vi "C-Scan - Reverse B-Scan.vi"(7 "Micropulse # In":i32, 8 "Define C-Scan Index":T1={"Index Start"=0.0, "Index Length"=260.0, "Indexing\nResolution"=5.0, "Ch1 Start"=0.0, "Ch1 Finish"=0.0, "Ch2 Start"=0.0, "Ch2 Finish"=0.0} {"Ch2 Finish" format="%#_6f"; "Ch2 Start" format="%#_6f"; "Ch1 Finish" format="%#_6f"; "Ch1 Start" format="%#_6f"; "Index Start" format="%#_6f"; "Index Length" format="%#_6f"; "Indexing\nResolution" format="%#_6f"}, 9 "FLZ Scan definition":T2={"Scan Start"=0.0, "Scan Length"=280.0, "Inspection Resolution"=0.5, "Direction"=enum."Forwards"} {"Inspection Resolution" format="%#_6f"; "Scan Start" format="%#_6f"; "Scan Length" format="%#_6f"}, 10 "C-Scan In Progress?":bool, 11 "B-Scan In Progress?":bool) -> (3 "B-Scan Just Finished?":bool)   [LabVIEW 2026, in "MicroPulse_Driver.lvlib"]
uses:
  MicroPulse_Driver.lvlib
  Data/Datatypes/MP - fly scan range.ctl
  Data/Datatypes/MP - inspection direction.ctl
  Data/Datatypes/MP - C-Scan Definition.ctl
  Low Level/FGV - B-Scan Active - Action [Enum].ctl
  <instrlib>/Micropulse/Micropulse.lvlib
panel:
  # "C-Scan Index"
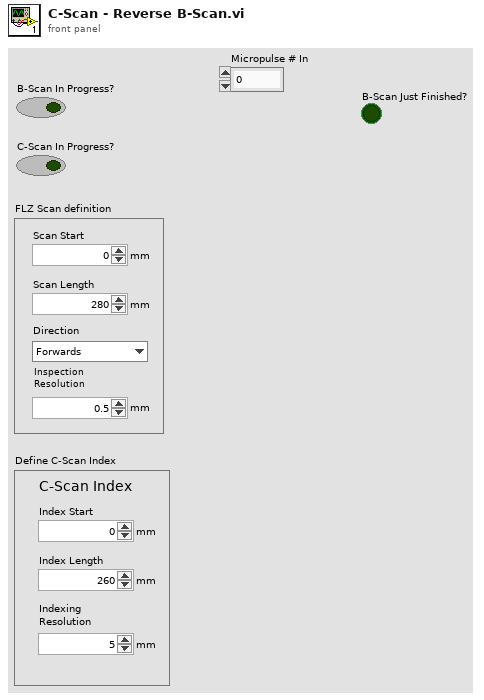
[diagram p1: front panel]
types:
  T1 = typedef "Micropulse.lvlib/MP - C-Scan Definition.ctl" = cluster{"Index Start":dbl, "Index Length":dbl, "Indexing\nResolution":dbl, "Ch1 Start":dbl, "Ch1 Finish":dbl, "Ch2 Start":dbl, "Ch2 Finish":dbl}
  T2 = typedef "Micropulse.lvlib/MP - fly scan range.ctl" = cluster{"Scan Start":dbl, "Scan Length":dbl, "Inspection Resolution":dbl, "Direction":T3}
  T3 = typedef "Micropulse.lvlib/MP - inspection direction.ctl" = enum16{"Forwards", "Backwards"}
  T4 = typedef "MicroPulse_Driver.lvlib/FGV - B-Scan Active - Action [Enum].ctl" = enum16{"Read", "Read & Reset Start Flag", "Start B-Scan", "B-Scan Finished"}
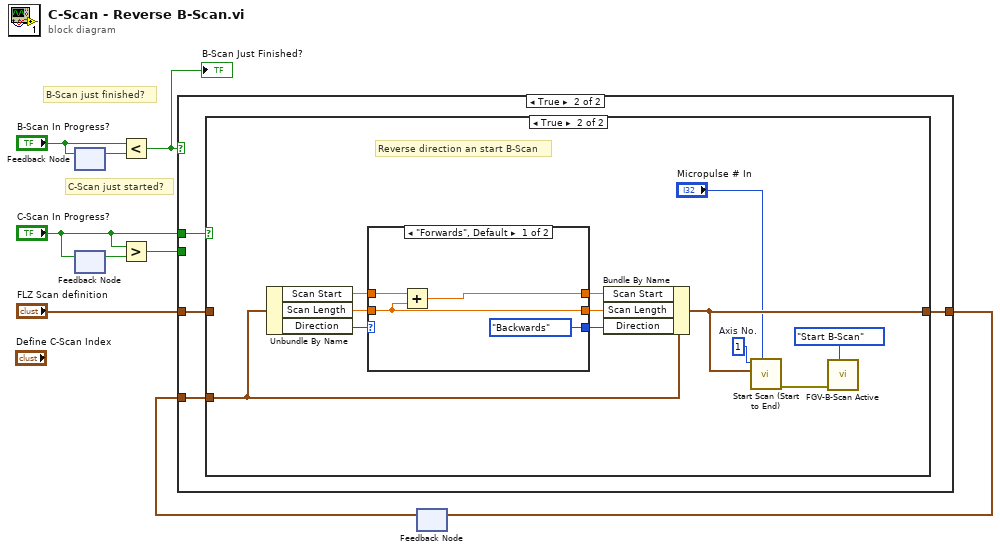
[diagram p0: block diagram]
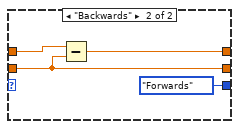
[diagram p5: hidden frame]
diagram:
  # "C-Scan just started?"
  # "B-Scan just finished?"
  n1 = feedback-in #1("B-Scan In Progress?") -> ()
  n2 = feedback #1() -> (w6:bool)  [unwired: 1 in]
  n3 = feedback #2() -> (w4:bool)  [unwired: 1 in]
  n4 = feedback-in #2("C-Scan In Progress?") -> ()
  n5 = Less?(x="B-Scan In Progress?", y=w6) -> (x < y?=w9:bool)
  "B-Scan Just Finished?" <- w9
  n6 = Greater?(x="C-Scan In Progress?", y=w4) -> (0:w5:bool)
  n7 = feedback #3() -> (w1:T2)  [unwired: 1 in]
  n8 = case shown="True" w9 {
    tunnel: "C-Scan In Progress?" -> [_ w19]
    tunnel: "FLZ Scan definition" -> [w12 w18]
    tunnel: w5 -> [w13 _]
    tunnel: [w11 w16] -> w2
    tunnel: w1 -> [w10 w17]
    frame False {
      n9 = case shown="False" w13 {
        tunnel: w12 -> [_ w15]
        tunnel: [w14 w15] -> w11
        tunnel: w10 -> [w14 _]
        frame False {
        }
        frame True {
          # "Save Scan Definition"
          # "C-Scan just started"
        }
      }
    }
    frame True {
      n10 = case shown="True" w19 {
        tunnel: w18 -> [_ _]
        tunnel: w17 -> [w20 w29]
        tunnel: [w20 w22] -> w16
        frame False {
        }
        frame True {
          w25 = u8 1  # Axis No.
          # "Reverse direction an start B-Scan"
          n11 = Unbundle By Name(w29) -> ("Scan Start"=w31:dbl, "Scan Length"=w30:dbl, "Direction"=w32:T3)
          n12 = case shown="\"Forwards\", Default" w32 {
            tunnel: w31 -> [w35 w39]
            tunnel: w30 -> [w33 w38]
            tunnel: [w34 w37] -> w28
            tunnel: [MP_-_inspection_direction."Backwards" ("Direction") MP_-_inspection_direction."Forwards" ("Direction")] -> w27
            tunnel: [w33 w38] -> w26
            frame "Forwards", Default {
              n13 = Add(x=w35, y=w33) -> (x+y=w34:dbl)
            }
            frame "Backwards" {
              n14 = Subtract(x=w39, y=w38) -> (x-y=w37:dbl)
            }
          }
          n15 = Bundle By Name(cluster=w29, "Scan Start"=w28, "Scan Length"=w26, "Direction"=w27) -> (w22:T2)
          n16 = call "Start Scan (Start to End).vi"("Micropulse # In"="Micropulse # In", "Scan definition"=w22, "Axis No."=w25) -> ("error out"=w24:errorcluster)  [unwired: 7 in, 1 out]
          n17 = call "FGV-B-Scan Active.vi"("Action"=FGV_-_B-Scan_Active_-_Action_[Enum]."Start B-Scan", "error in (no error)"=w24) -> ()  [unwired: 7 in, 3 out]
        }
      }
    }
  }
  n18 = feedback-in #3(w2) -> ()
